vi "LJStreamM.vi"() -> ()   [LabVIEW 2026]
uses:
  Common Logger Controls/Currently Opened Device Params.ctl
  Common Logger Controls/Device Open Config Cluster.ctl
  Common Logger Controls/Channel Setup.ctl
  Common Logger Controls/Row Modification Options.ctl
  Common Logger Controls/Program Config Cluster.ctl
  sub/LJStreamM Front Panel References.ctl
  Common Logger VIs/LJM logger Globals.vi
panel:
  in  "Channel Setup":T1={"Name"=["AIN0", "AIN1", "AIN2", "AIN3", "AIN4", "AIN5", "AIN6", "AIN7", "AIN8", "AIN9", "AIN10", "AIN11", "AIN12", "AIN13", "AIN14", "AIN15", "AIN16", "AIN17", "AIN18", "AIN19", "AIN20", "AIN21", "AIN22", "AIN23", "AIN24", "AIN25", "AIN26", "AIN27", "AIN28", "AIN29", "AIN30", "AIN31", "AIN32", "AIN33", "AIN34", "AIN35", "AIN36", "AIN37", "AIN38", "AIN39", "AIN40", "AIN41", "AIN42", "AIN43", "AIN44", "AIN45", "AIN46", "AIN47", "AIN48", "AIN49", "AIN50", "AIN51", "AIN52", "AIN53", "AIN54", "AIN55", "AIN56", "AIN57", "AIN58", "AIN59", "AIN60", "AIN61", "AIN62", "AIN63", "AIN64", "AIN65", "AIN66", "AIN67", "AIN68", "AIN69", "AIN70", "AIN71", "AIN72", "AIN73", "AIN74", "AIN75", "AIN76", "AIN77", "AIN78", "AIN79", "AIN80", "AIN81", "AIN82", "AIN83", "AIN84", "AIN85", "AIN86", "AIN87", "AIN88", "AIN89", "AIN90", "AIN91", "AIN92", "AIN93", "AIN94", "AIN95", "AIN96", "AIN97", "AIN98", "AIN99"], "", "Scaling Equation"=["y=a", "y=b", "y=c", "y=d", "y=e", "y=f", "y=g", "y=h", "y=i", "y=j", "y=k", "y=l", "y=m", "y=n", "y=o", "y=p", "y=q", "y=r", "y=s", "y=t", "y=u", "y=v", "y=w", "y=x", "y=y", "y=z", "y=a2", "y=b2", "y=c2", "y=d2", "y=e2", "y=f2", "y=g2", "y=h2", "y=i2", "y=j2", "y=k2", "y=l2", "y=m2", "y=n2", "y=o2", "y=p2", "y=q2", "y=r2", "y=s2", "y=t2", "y=u2", "y=v2", "y=w2", "y=x2", "y=y2", "y=z2", "y=a3", "y=b3", "y=c3", "y=d3", "y=e3", "y=f3", "y=g3", "y=h3", "y=i3", "y=j3", "y=k3", "y=l3", "y=m3", "y=n3", "y=o3", "y=p3", "y=q3", "y=r3", "y=s3", "y=t3", "y=u3", "y=v3", "y=w3", "y=x3", "y=y3", "y=z3", "y=a4", "y=b4", "y=c4", "y=d4", "y=e4", "y=f4", "y=g4", "y=h4", "y=i4", "y=j4", "y=k4", "y=l4", "y=m4", "y=n4", "y=o4", "y=p4", "y=q4", "y=r4", "y=s4", "y=t4", "y=u4", "y=v4"], "", "Graph?"=[TRUE, TRUE, TRUE, TRUE, FALSE, FALSE, FALSE, FALSE, FALSE, FALSE, FALSE, FALSE, FALSE, FALSE, FALSE, FALSE]}
  in  "Stop Stream":bool
  out "Open Configs":T2
  out "Currently Opened Device Params":T3={"Device Type"="ANY", "Connection Type"="ANY", "Serial Number"=0}
  out "Program Config Name":string
  out "Open Config Name":string
  in  "Configuration":bool
  out "LJMScanBacklog":dbl format="%.2f"
  out "DeviceScanBacklog":dbl format="%.2f"
  in  "Disable Scaling*":bool=TRUE
  out "ms Per Loop":u32
  out "Scans Per Iteration":u32
  out "Iteration Number":i32
  out "Last Command-Response Error Message":string="No Error"
  in  "Max File Size (Bytes)":i32=1048576 min=1 max=2000000000
  out "Scaled Value":dbl[](array[numeric]) format="%.6f"
  out "Raw Value":dbl[](array[numeric]) format="%.6f"
  in  "Log To File":bool
  in  "exit":bool
  in  "# Scans On Graph":i32=1000 min=0
  in  "# Channels":i32=1 min=1 max=96
  out "Waveform Graph":cluster{dbl, dbl, dbl[][]}(graph)={0.0, 0.0025, []}
  in  "Scan Rate (Hz)":dbl=100.0 format="%.3f"
  out "Current Data File":path=path "Not Logging To File"
  in  "Data File Prefix":string="data"
  in  "start stream":bool caption="Start Stream"
  out "Last Stream Error Message":string="No Error"
  out "App Name":string
  in  "Row Modification Options":T4 {"Row #" min=0 max=95}
  # "Graph?"
  # "Name"
  # "Raw Value"
  # "Scaling Equation"
  # "Scaled Value"
  # "The raw value for each row corresponds to a scaling variable:"
  # "row 0-15   -->  \"a\"-\"p\""
  # "row 16-31 -->  \"a2\"-\"p2\""
  # "row 32-47 -->  \"a3\"-\"p3\""
  # "row 48-63 -->  \"a4\"-\"p4\""
  # "row 64-79 -->  \"a5\"-\"p5\""
  # "row 80-96 -->  \"a6\"-\"p6\""
  # "The scaled value for a row is represented by the variable  \"y\" in the row's scaling equation."
  # "If your scaling  equation has an error, the scaled value will be zero."
  # "*Scaling is computing intensive. If the LJM Backlog is growing, disable scaling."
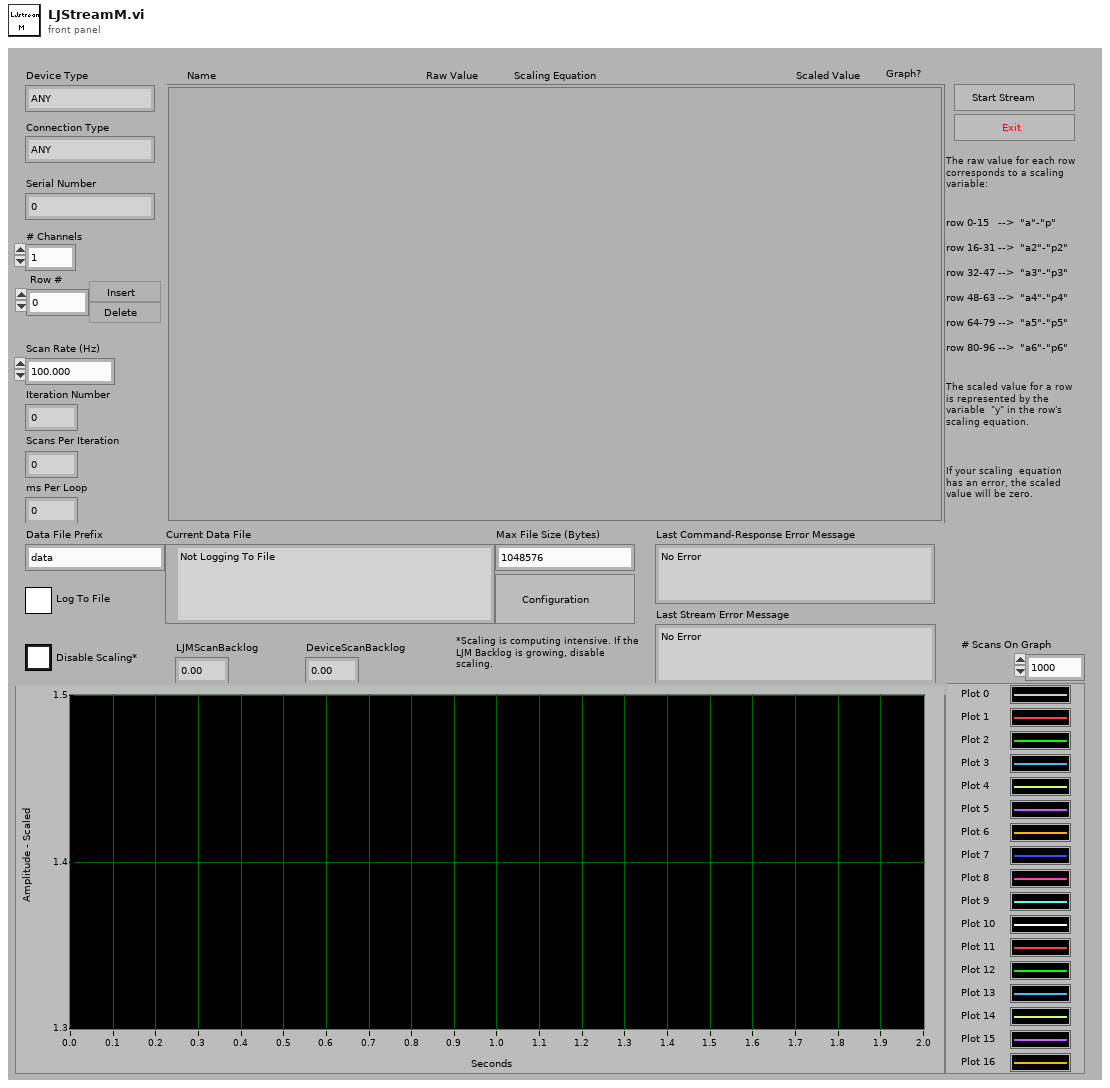
[diagram p1: front panel]
types:
  T1 = typedef "Channel Setup.ctl" = cluster{"Name":string[], string, "Scaling Equation":string[], string, "Graph?":bool[]}
  T2 = typedef "Device Open Config Cluster.ctl" = cluster{"Open Config Device Type":string, "Open Config Connection Type":string, "Open Config Identifier":string}
  T3 = typedef "Currently Opened Device Params.ctl" = cluster{"Device Type":string, "Connection Type":string, "Serial Number":i32}
  T4 = typedef "Row Modification Options.ctl" = cluster{" Row #":i32, "Delete Row":bool, "Insert Row":bool}
  T5 = typedef "LJStreamM Front Panel References.ctl" = cluster{"# Scans Read":refnum<vi>, "# of iterations Ref":refnum<vi>, "ms Per Loop Ref":refnum<vi>, "DeviceScanBacklog Ref":refnum<vi>, "LJMScanBacklog Ref":refnum<vi>, "Stop Stream Ref":refnum<vi>, "Disable Scaling* Ref":refnum<vi>, "Write To File Ref":refnum<vi>, "Current Data File Ref":refnum<vi>, "Waveform Graph Ref":refnum<vi>, "Data File Prefix Ref":refnum<vi>, "Max File Size (Bytes) Ref":refnum<vi>, "Channel Setup Reference In":refnum<vi>}
  T6 = typedef "Program Config Cluster.ctl" = cluster{"Data File Prefix":string, "Scan Rate (Hz)":dbl, "Graph History":i32, "# Channels":i32, "Disable Scaling":bool, "Max File Size (Bytes)":i32, "Channel Setup":T1, "Interval (ms)":u32, "Write To File":bool, "Log Every n Scans":i32}
  T7 = enum16{"Initialization", "Data Acquisition", "Shutdown", "Reconfiguration"}
  T8 = cluster{"Name":string[], string, "Scaling Equation":string[], string, "Graph?":bool[]}
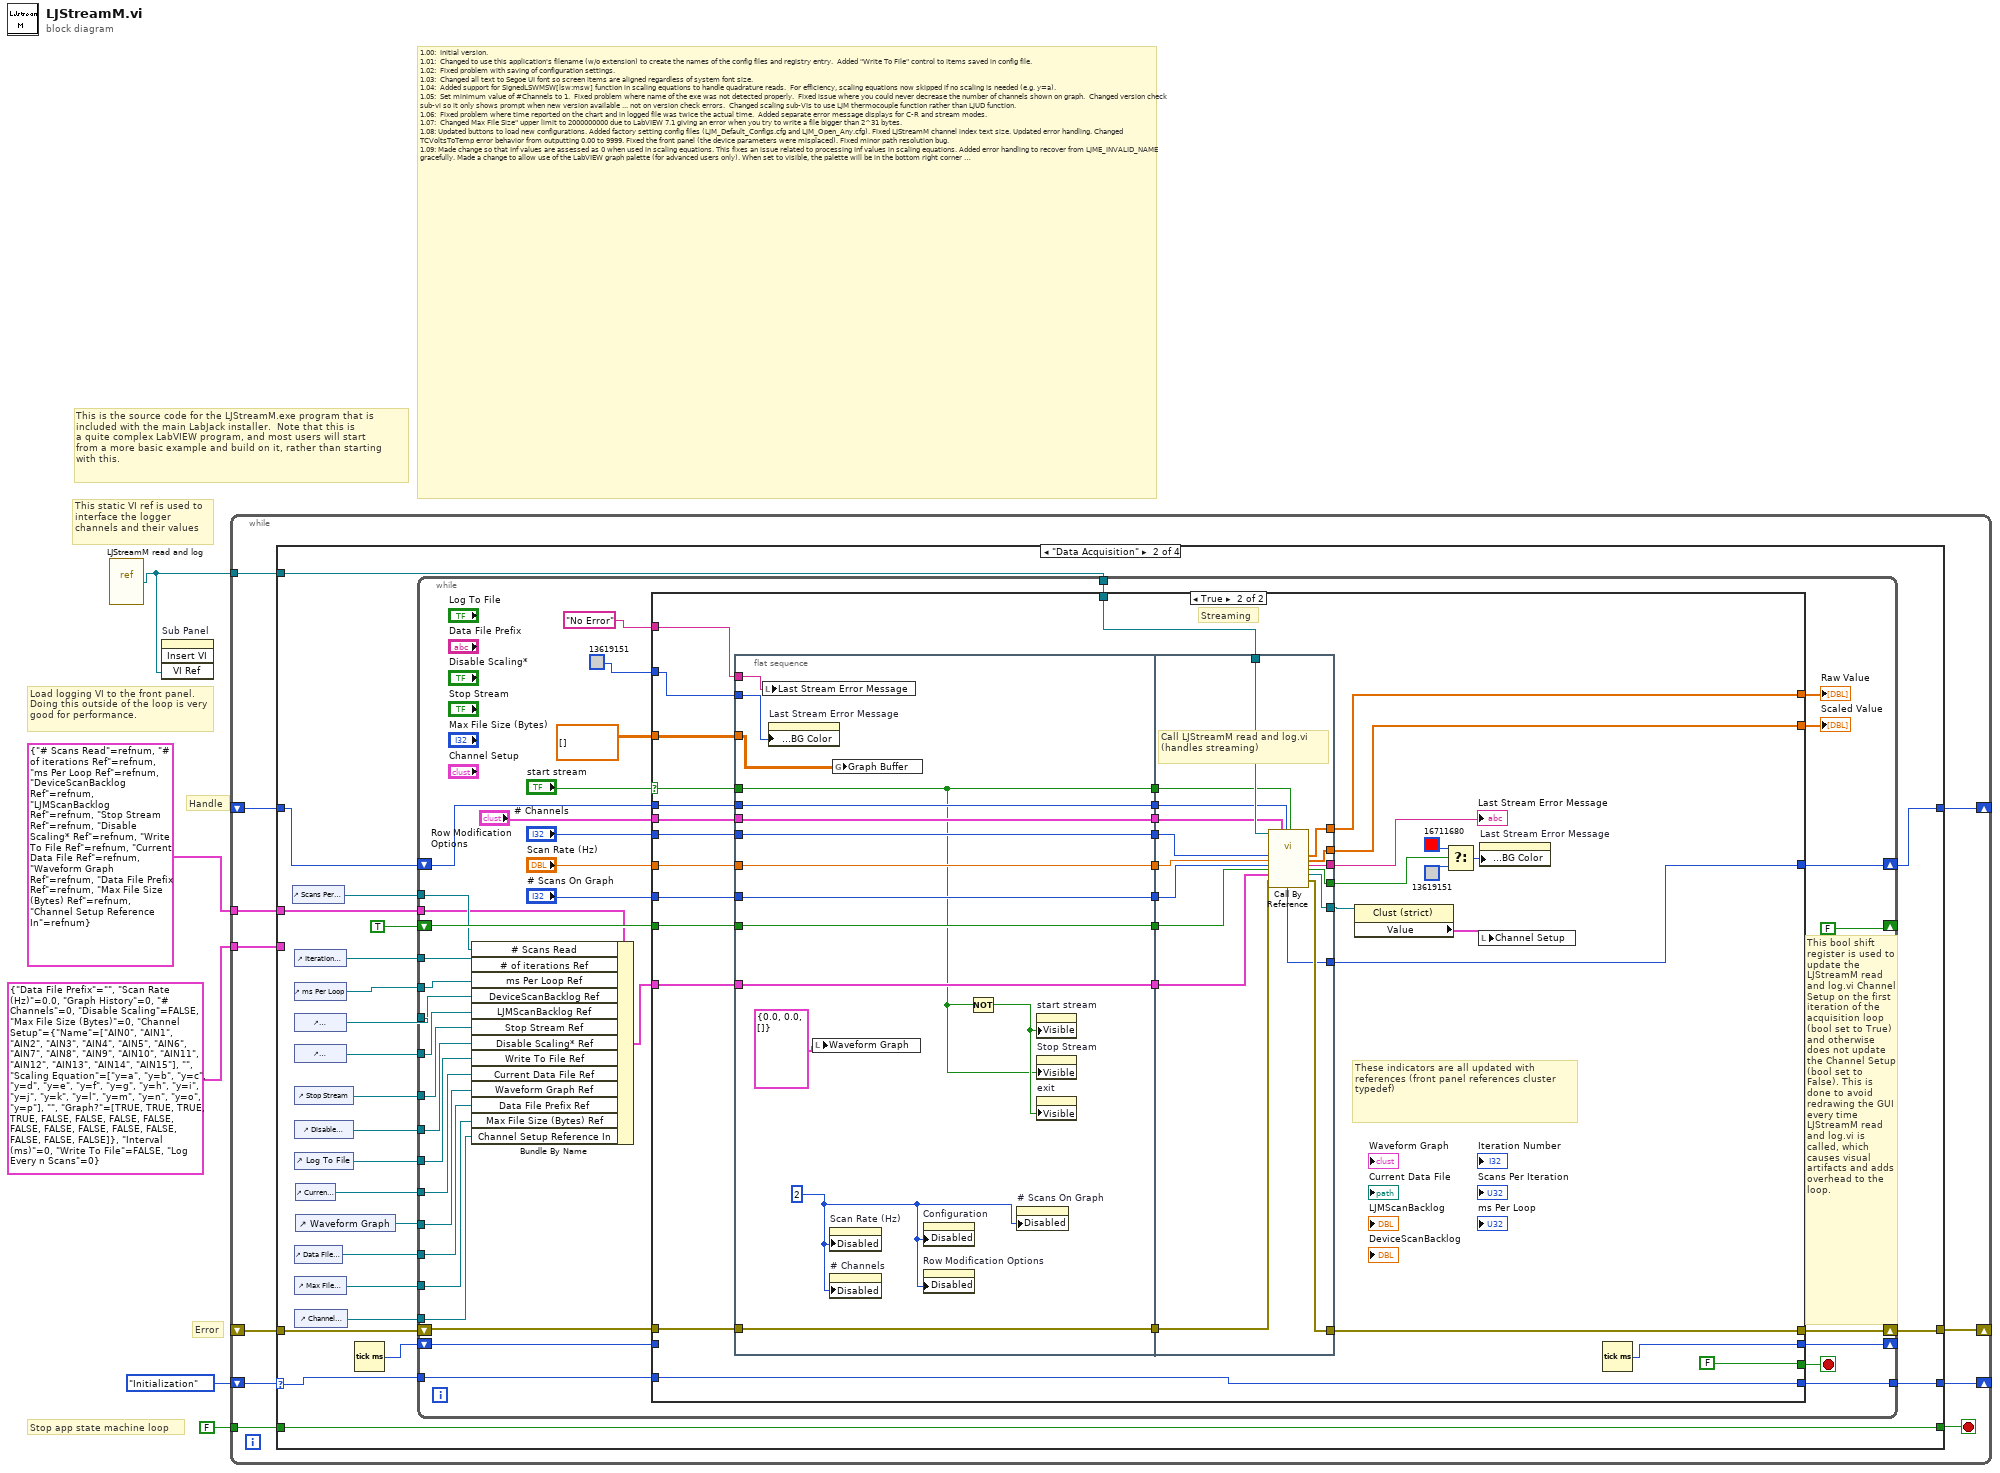
[diagram p0: block diagram]
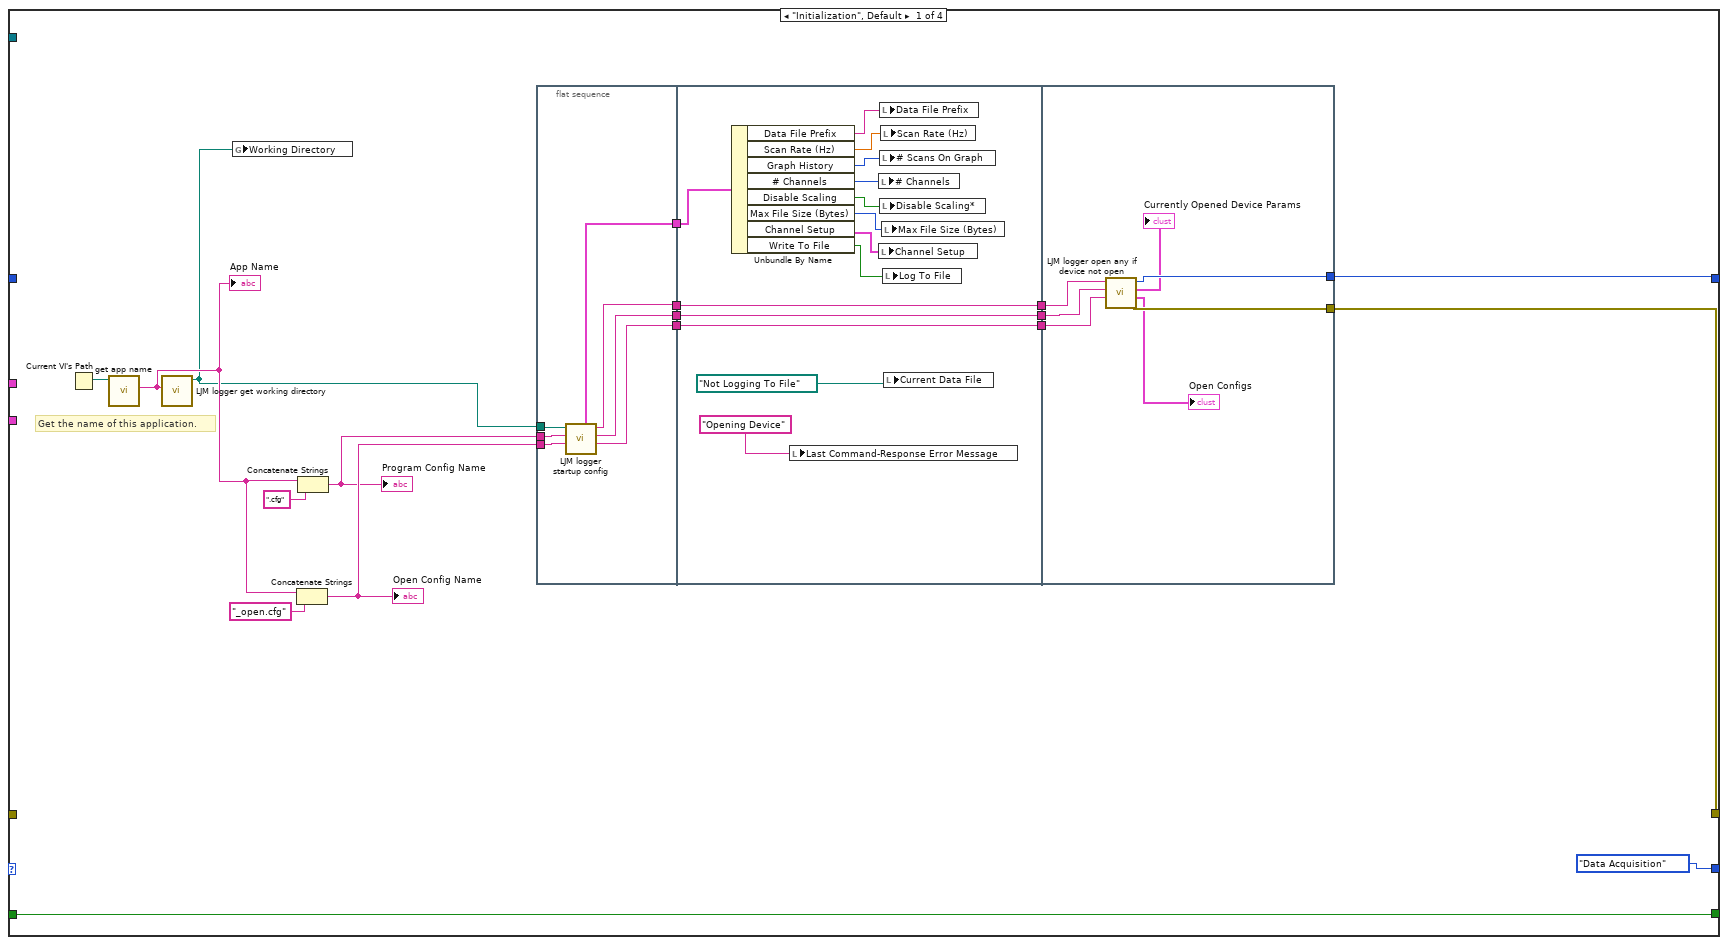
[diagram p2: hidden frame]
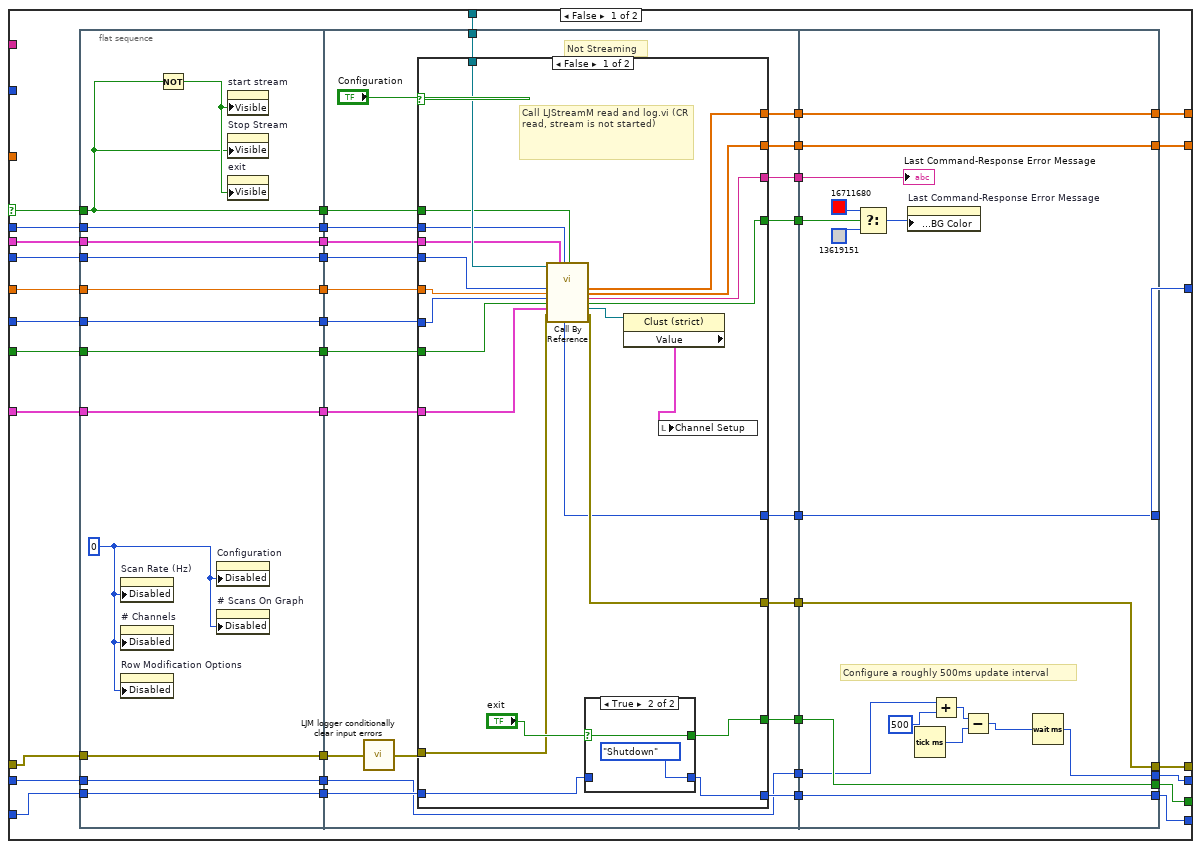
[diagram p3: hidden frame]
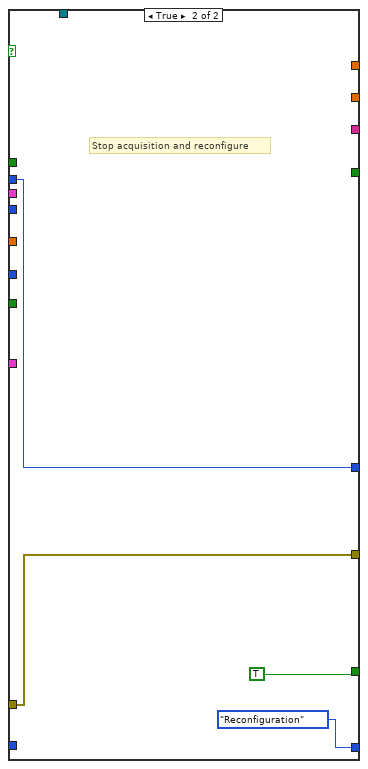
[diagram p5: hidden frame]
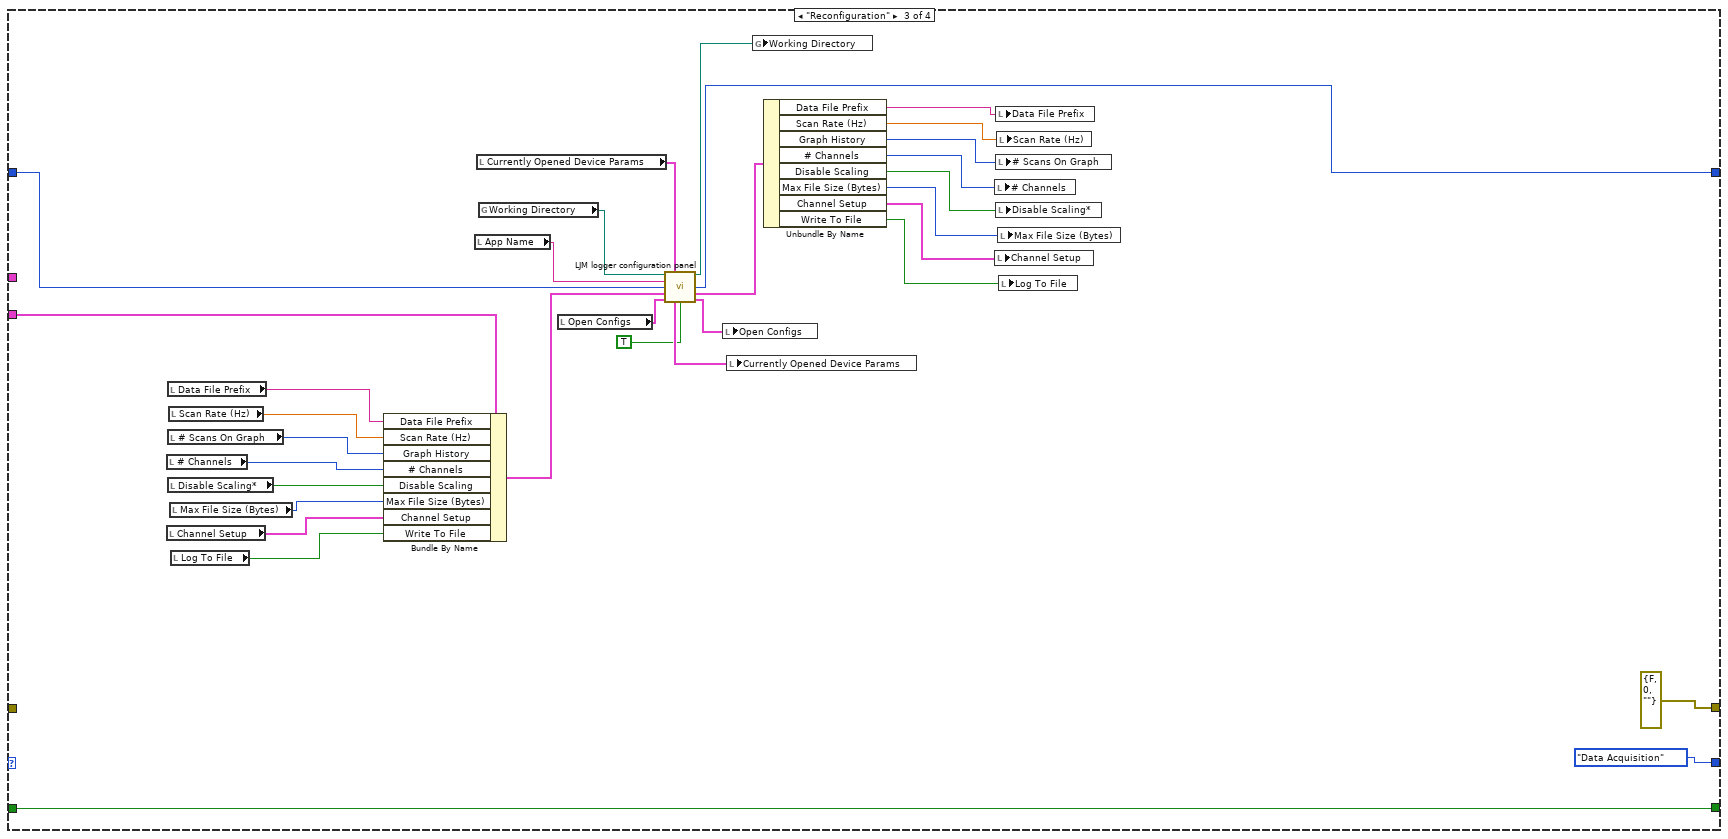
[diagram p6: hidden frame]
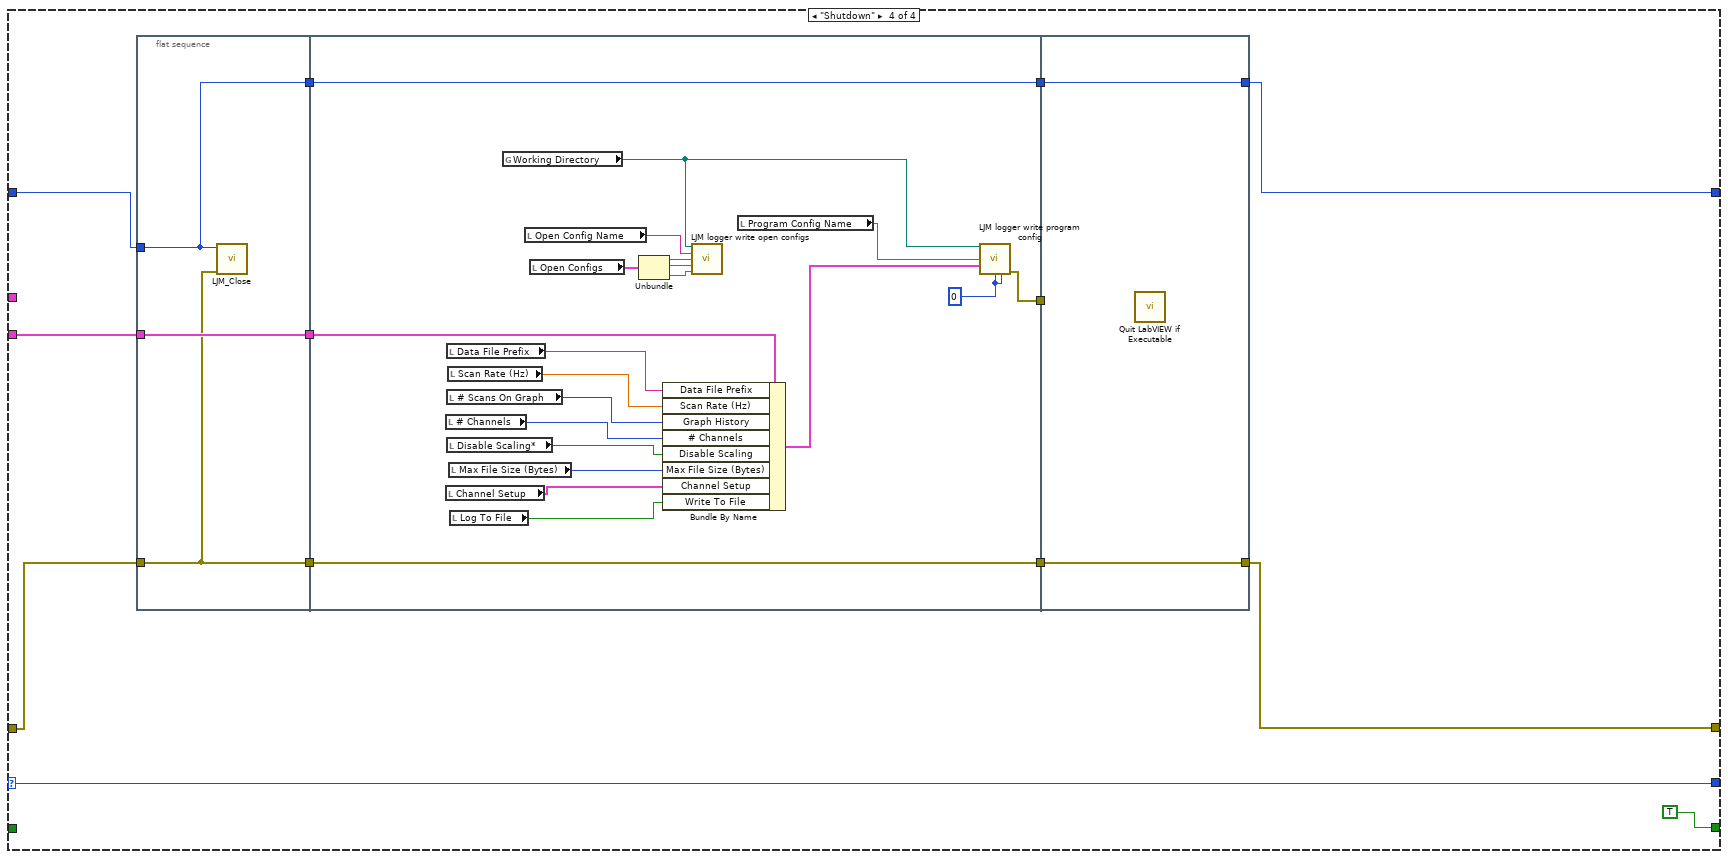
[diagram p7: hidden frame]
diagram:
  # "This static VI ref is used to interface the logger channels and their values"
  # "Load logging VI to the front panel. Doing this outside of the loop is very good for performance."
  # "Stop app state machine loop"
  # "Error"
  # "Handle"
  # "This is the source code for the LJStreamM.exe program that is\nincluded with the main LabJack installer.  Note that this is \na quite complex LabVIEW program, and most users will start\nfrom a more basic example and build on it, rather than starting\nwith this."
  # "1.00:  Initial version.\n1.01:  Changed to use this application's filename (w/o extension) to create the names of the config files and registry entry.  Added \"Write To File\" control to items saved in config file.\n1.02:  Fixed problem with saving of configuration settings.\n1.03:  Changed all text to Segoe UI font so screen items are aligned regardless of system font size.\n1.04:  Added support for SignedLSWMSW[lsw:msw] function in scaling equations to handle quadrature reads.  For efficiency, scaling equations now skipped if no scaling is needed (e.g. y=a).\n1.05:  Set minimum value of #Channels to 1.  Fixed problem where name of the exe was not detected properly.  Fixed issue where you could never decrease the number of channels shown on graph.  Changed version check sub-vi so it only shows prompt when new version available ... not on version check errors.  Changed scaling sub-VIs to use LJM thermocouple function rather than LJUD function.\n1.06:  Fixed problem where time reported on the chart and in logged file was twice the actual time.  Added separate error message displays for C-R and stream modes.\n1.07:  Changed Max File Size\" upper limit to 2000000000 due to LabVIEW 7.1 giving an error when you try to write a file bigger than 2^31 bytes.\n1.08: Updated buttons to load new configurations. Added factory setting config files (LJM_Default_Configs.cfg and LJM_Open_Any.cfg). Fixed LJStreamM channel index text size. Updated error handling. Changed TCVoltsToTemp error behavior from outputting 0.00 to 9999. Fixed the front panel (the device parameters were misplaced). Fixed minor path resolution bug.\n1.09: Made change so that Inf values are assessed as 0 when used in scaling equations. This fixes an issue related to processing Inf values in scaling equations. Added error handling to recover from LJME_INVALID_NAME gracefully. Made a change to allow use of the LabVIEW graph palette (for advanced users only). When set to visible, the palette will be in the bottom right corner of the LJStreamM graph. \n1.10: Fixed SignedMSWLSW scaling equation functionality. This was previously returning an unsigned 32-bit integer representation. It now returns a signed 32-bit integer representation.\n1.11: Reworked configs including adding a config panel. Moved 'Change Working Directory'. Refactored write to file functionality. Refactored diagram. Added scaling equation error messaging. Renamed 'experiment' config 'program' config. Added register write functionality to configuration panel. Increased front panel text size, changed font to Arial (monospace), and set the minimum panel size. Added support for 96 channels.  Added logger row modification controls. Note: program configs with 96 channels in v1.11 would not be recognized as valid in v1.10.\n1.12: Made minor Visual tweaks to the front panel. Made optimizations to scaling equation processing and front panel responsiveness. Disabled the scaling equation control while stream is active.\n1.13: If a config file does not exist, load defaults without warning the user. Usually if the config file does not exist it means this is the first time running the program, and we do not want new users to see a warning about the config not existing. Rearranged logger graph palettes on the front panel"
  n1 = vi-ref "LJStreamM read and log.vi"() -> ("vi reference"=w2:refnum<vi>)
  n2 = invoke on="Sub Panel" class="SubPanel" method="Insert VI"("VI Ref"=w2) -> ()  [unwired: 3 in, 4 out]
  n3 = while {
    shift-right: [w14] -> _
    shift-left: _ -> [w11]
    shift-right: [w15] -> _
    shift-left: _ -> [w12]
    shift-right: [w13] -> _
    shift-left: T7."Initialization" -> [w16]
    tunnel: T6 {"Data File Prefix"="", "Scan Rate (Hz)"=0.0, "Graph History"=0, "# Channels"=0, "Disable Scaling"=FALSE, "Max File Size (Bytes)"=0, "Channel Setup"={"Name"=["AIN0", "AIN1", "AIN2", "AIN3", "AIN4", "AIN5", "AIN6", "AIN7", "AIN8", "AIN9", "AIN10", "AIN11", "AIN12", "AIN13", "AIN14", "AIN15"], "", "Scaling Equation"=["y=a", "y=b", "y=c", "y=d", "y=e", "y=f", "y=g", "y=h", "y=i", "y=j", "y=k", "y=l", "y=m", "y=n", "y=o", "y=p"], "", "Graph?"=[TRUE, TRUE, TRUE, TRUE, FALSE, FALSE, FALSE, FALSE, FALSE, FALSE, FALSE, FALSE, FALSE, FALSE, FALSE, FALSE]}, "Interval (ms)"=0, "Write To File"=FALSE, "Log Every n Scans"=0} ("Program Configs") -> [w10]
    tunnel: FALSE -> [w8]
    tunnel: w2 -> [w7]
    tunnel: T5 {"# Scans Read"=refnum, "# of iterations Ref"=refnum, "ms Per Loop Ref"=refnum, "DeviceScanBacklog Ref"=refnum, "LJMScanBacklog Ref"=refnum, "Stop Stream Ref"=refnum, "Disable Scaling* Ref"=refnum, "Write To File Ref"=refnum, "Current Data File Ref"=refnum, "Waveform Graph Ref"=refnum, "Data File Prefix Ref"=refnum, "Max File Size (Bytes) Ref"=refnum, "Channel Setup Reference In"=refnum} ("LJStreamM Front Panel References") -> [w6]
    stop <- w9 stop-if-true
    n4 = case shown="\"Data Acquisition\"" w16 {
      selector: w16 -> [_ w69 _ w357]
      tunnel: [w20 w84 w343 w347] -> w15
      tunnel: [w19 w83 errorcluster {"status"=FALSE, "code"=0, "source"=""} ("error out") w346] -> w14
      tunnel: [T7."Data Acquisition" w85 T7."Data Acquisition" w357] -> w13
      tunnel: w12 -> [_ w81 w342 w353]
      tunnel: w11 -> [_ w82 _ w352]
      tunnel: w10 -> [_ _ w340 w356]
      tunnel: [w17 w86 w339 TRUE] -> w9
      tunnel: w8 -> [w17 w86 w339 _]
      tunnel: w7 -> [_ w80 _ _]
      tunnel: w6 -> [_ w68 _ _]
      frame "Initialization", Default {
        # "Get the name of this application."
        n5 = Current VI's Path() -> (path=w21:path)
        n6 = call "get app name.vi"("Current VI's Path"=w21) -> ("App Name Without Extension"=w25:string)  [unwired: 4 in, 2 out]
        "App Name" <- w25
        n7 = call "LJM logger get working directory.vi"("Application Name"=w25) -> ("Working Directory"=w22:path)  [unwired: 9 in, 1 out]
        n8 = global write "LJM logger Globals.vi" "Working Directory"(w22) -> ()
        n9 = Concatenate Strings(w25, "_open.cfg" ("string")) -> (w27:string)
        "Open Config Name" <- w27
        n10 = Concatenate Strings(w25, ".cfg" ("string")) -> (w26:string)
        "Program Config Name" <- w26
        n11 = flat-sequence {
          tunnel: [w40] -> w34
          tunnel: [w39] -> w33
          tunnel: [w38] -> w32
          tunnel: w22 -> [w41]
          tunnel: w26 -> [w37]
          tunnel: w27 -> [w36]
          tunnel: [w35] -> w31
          tunnel: w34 -> [w55]
          tunnel: w33 -> [w54]
          tunnel: w32 -> [w53]
          tunnel: [w55] -> w30
          tunnel: [w54] -> w29
          tunnel: [w53] -> w28
          tunnel: w31 -> [w52]
          tunnel: w30 -> [w62]
          tunnel: w29 -> [w61]
          tunnel: w28 -> [w60]
          tunnel: [w58] -> w19
          tunnel: [w59] -> w20
          frame #0 {
            n12 = call "LJM logger startup config.vi"("Device Open Config Name"=w36, "Program Config Name"=w37, "Working Directory"=w41) -> ("Open Config Identifier"=w38:string, "Open Config ConnectionType"=w39:string, "Open Config Device Type"=w40:string, "Program Configs"=w35:T6)  [unwired: 3 in]
          }
          frame #1 {
            n13 = Unbundle By Name(w52) -> ("Data File Prefix"=w51:string, "Scan Rate (Hz)"=w50:dbl, "Graph History"=w49:i32, "# Channels"=w48:i32, "Disable Scaling"=w47:bool, "Max File Size (Bytes)"=w46:i32, "Channel Setup"=w44:T1, "Write To File"=w45:bool)
            n14 = local write "Last Command-Response Error Message"("Opening Device" ("source")) -> ()
            n15 = local write "# Channels"(w48) -> ()
            n16 = local write "Channel Setup"(w44) -> ()
            n17 = local write "Data File Prefix"(w51) -> ()
            n18 = local write "# Scans On Graph"(w49) -> ()
            n19 = local write "Disable Scaling*"(w47) -> ()
            n20 = local write "Scan Rate (Hz)"(w50) -> ()
            n21 = local write "Max File Size (Bytes)"(w46) -> ()
            n22 = local write "Log To File"(w45) -> ()
            n23 = local write "Current Data File"(path "Not Logging To File" ("Current Data File")) -> ()
          }
          frame #2 {
            n24 = call "LJM logger open any if device not open.vi"("Open Config Identifier"=w60, "Open Config Connection Type"=w61, "Open Config DeviceType"=w62) -> ("error out"=w58:errorcluster, "Open Configs"=→"Open Configs":T2, "Currently Opened Device Params"=→"Currently Opened Device Params":T3, "Handle Out"=w59:i32)  [unwired: 5 in]
          }
        }
      }
      frame "Data Acquisition" {
        n25 = control-ref of="Scans Per Iteration"() -> (w79:refnum<vi>)
        n26 = control-ref of="Iteration Number"() -> (w78:refnum<vi>)
        n27 = control-ref of="ms Per Loop"() -> (w77:refnum<vi>)
        n28 = control-ref of="DeviceScanBacklog"() -> (w76:refnum<vi>)
        n29 = control-ref of="LJMScanBacklog"() -> (w75:refnum<vi>)
        n30 = control-ref of="Stop Stream"() -> (w74:refnum<vi>)
        n31 = control-ref of="Disable Scaling*"() -> (w73:refnum<vi>)
        n32 = control-ref of="Log To File"() -> (w72:refnum<vi>)
        n33 = control-ref of="Data File Prefix"() -> (w67:refnum<vi>)
        n34 = control-ref of="Max File Size (Bytes)"() -> (w66:refnum<vi>)
        n35 = control-ref of="Channel Setup"() -> (w65:refnum<vi>)
        n36 = control-ref of="Current Data File"() -> (w71:refnum<vi>)
        n37 = control-ref of="Waveform Graph"() -> (w70:refnum<vi>)
        n38 = Tick Count (ms)() -> (millisecond timer value=w63:u32)
        n39 = while {
          shift-right: [w93] -> w84
          shift-left: w81 -> [w110]
          shift-right: [w114] -> w83
          shift-left: w82 -> [w111]
          tunnel: w80 -> [w116]
          shift-right: [FALSE] -> _
          shift-left: TRUE -> [w115]
          tunnel: [w108] -> w85
          tunnel: w79 -> [w106]
          tunnel: w78 -> [w105]
          tunnel: w77 -> [w104]
          tunnel: w76 -> [w103]
          tunnel: w75 -> [w102]
          tunnel: w74 -> [w101]
          tunnel: w73 -> [w100]
          tunnel: w72 -> [w99]
          tunnel: w71 -> [w98]
          tunnel: w70 -> [w97]
          tunnel: w69 -> [w109]
          tunnel: w68 -> [w96]
          tunnel: w67 -> [w95]
          tunnel: w66 -> [w94]
          tunnel: w65 -> [w91]
          shift-right: [w88] -> _
          shift-left: w63 -> [w87]
          stop <- w107 stop-if-true
          # "This bool shift register is used to update the LJStreamM read and log.vi Channel Setup on the first iteration of the acquisition loop (bool set to True) and otherwise does not update the Channel Setup (bool set to False). This is done to avoid redrawing the GUI every time LJStreamM read and log.vi is called, which causes visual artifacts and adds overhead to the loop."
          n40 = Bundle By Name(cluster=w96, "# Scans Read"=w106, "# of iterations Ref"=w105, "ms Per Loop Ref"=w104, "DeviceScanBacklog Ref"=w103, "LJMScanBacklog Ref"=w102, "Stop Stream Ref"=w101, "Disable Scaling* Ref"=w100, "Write To File Ref"=w99, "Current Data File Ref"=w98, "Waveform Graph Ref"=w97, "Data File Prefix Ref"=w95, "Max File Size (Bytes) Ref"=w94, "Channel Setup Reference In"=w91) -> (w92:T5)
          n41 = case shown="True" "start stream" {
            selector: "start stream" -> [w157 w272]
            tunnel: dbl[][] [] ("Graph Buffer") -> [_ w253]
            tunnel: u32 13619151 -> [_ w254]
            tunnel: "No Error" ("Last Stream Error Message") -> [_ w255]
            tunnel: "# Scans On Graph" -> [w161 w276]
            tunnel: "# Channels" -> [w159 w274]
            tunnel: "Scan Rate (Hz)" -> [w160 w275]
            tunnel: w116 -> [w162 w256]
            tunnel: w115 -> [w153 w268]
            tunnel: w110 -> [w158 w273]
            tunnel: w111 -> [w155 w277]
            tunnel: [w156 w271] -> w114
            tunnel: [w135 w267] -> w113
            tunnel: [w137 w266] -> w112
            tunnel: [w154 w264] -> w108
            tunnel: w109 -> [w152 w264]
            tunnel: [w151 FALSE] -> w107
            tunnel: [w130 w250] -> w93
            tunnel: w92 -> [w139 w248]
            tunnel: "Row Modification Options" -> [w129 w247]
            tunnel: [w127 w245] -> w88
            tunnel: w87 -> [w124 _]
            frame False {
              n42 = flat-sequence {
                tunnel: w152 -> [w169]
                tunnel: w153 -> [w170]
                tunnel: w155 -> [w171]
                tunnel: w157 -> [w165]
                tunnel: w158 -> [w172]
                tunnel: w159 -> [w173]
                tunnel: w160 -> [w174]
                tunnel: w161 -> [w175]
                tunnel: [w175] -> w147
                tunnel: [w174] -> w146
                tunnel: [w173] -> w145
                tunnel: [w172] -> w144
                tunnel: [w165] -> w143
                tunnel: [w171] -> w142
                tunnel: [w170] -> w141
                tunnel: [w169] -> w140
                tunnel: w139 -> [w168]
                tunnel: [w168] -> w138
                tunnel: w129 -> [w167]
                tunnel: [w167] -> w128
                tunnel: w124 -> [w163]
                tunnel: [w163] -> w125
                tunnel: w162 -> [w197]
                tunnel: [w190] -> w150
                tunnel: [w187] -> w149
                tunnel: [w184] -> w148
                tunnel: w147 -> [w195]
                tunnel: w146 -> [w194]
                tunnel: w145 -> [w193]
                tunnel: w144 -> [w192]
                tunnel: w143 -> [w191]
                tunnel: w142 -> [w189]
                tunnel: w141 -> [w186]
                tunnel: w140 -> [w185]
                tunnel: w138 -> [w183]
                tunnel: [w182] -> w136
                tunnel: [w181] -> w134
                tunnel: [w180] -> w133
                tunnel: [w179] -> w132
                tunnel: [w178] -> w131
                tunnel: w128 -> [w177]
                tunnel: w125 -> [w176]
                tunnel: [w176] -> w126
                tunnel: [w242] -> w151
                tunnel: [w243] -> w154
                tunnel: [w244] -> w156
                tunnel: w150 -> [w244]
                tunnel: w149 -> [w243]
                tunnel: w148 -> [w242]
                tunnel: [w238] -> w137
                tunnel: w136 -> [w238]
                tunnel: [w237] -> w135
                tunnel: w134 -> [w237]
                tunnel: w133 -> [w236]
                tunnel: w132 -> [w235]
                tunnel: w131 -> [w234]
                tunnel: [w234] -> w130
                tunnel: [w233] -> w127
                tunnel: w126 -> [w228]
                frame #0 {
                  w164 = u8 0 ("Disabled")
                  n43 = property on="Scan Rate (Hz)" class="DigNum (strict)"("Disabled"=w164) -> ()  [unwired: 2 in, 2 out]
                  n44 = property on="# Channels" class="DigNum (strict)"("Disabled"=w164) -> ()  [unwired: 2 in, 2 out]
                  n45 = property on="Row Modification Options" class="Clust"("Disabled"=w164) -> ()  [unwired: 2 in, 2 out]
                  n46 = Not(x=w165) -> (.not. x?=w166:bool)
                  n47 = property on="Configuration" class="Bool"("Disabled"=w164) -> ()  [unwired: 2 in, 2 out]
                  n48 = property on="# Scans On Graph" class="DigNum (strict)"("Disabled"=w164) -> ()  [unwired: 2 in, 2 out]
                  n49 = property on="start stream" class="Bool"("Visible"=w166) -> ()  [unwired: 2 in, 2 out]
                  n50 = property on="Stop Stream" class="Bool (strict)"("Visible"=w165) -> ()  [unwired: 2 in, 2 out]
                  n51 = property on="exit" class="Bool"("Visible"=w166) -> ()  [unwired: 2 in, 2 out]
                }
                frame #1 {
                  # "Not Streaming"
                  n52 = call "LJM logger conditionally clear input errors.vi"("error in"=w189) -> ("error out"=w188:errorcluster)
                  n53 = case shown="False" "Configuration" {
                    tunnel: [w217 T7."Reconfiguration"] -> w187
                    tunnel: w197 -> [w214 _]
                    tunnel: w188 -> [w207 w226]
                    tunnel: [w201 w226] -> w190
                    tunnel: w186 -> [w199 _]
                    tunnel: w195 -> [w209 _]
                    tunnel: w194 -> [w210 _]
                    tunnel: w193 -> [w211 _]
                    tunnel: w192 -> [w212 w224]
                    tunnel: w191 -> [w213 _]
                    tunnel: w185 -> [w218 _]
                    tunnel: [w216 TRUE] -> w184
                    tunnel: w183 -> [w208 _]
                    tunnel: [w206 _] -> w182
                    tunnel: [w205 _] -> w181
                    tunnel: [w204 _] -> w180
                    tunnel: [w203 _] -> w179
                    tunnel: [w200 w224] -> w178
                    tunnel: w177 -> [w198 _]
                    frame False {
                      # "Call LJStreamM read and log.vi (CR read, stream is not started)"
                      n54 = call-by-ref "?"(reference=w214, "# Channels"=w211, "Scan Rate (Hz)"=w210, "# Scans On Graph"=w209, "Update Channel Ref"=w199, "LJStreamM Front Panel References"=w208, "(LJM) Error In"=w207, "Row Modification Options"=w198, "Handle In"=w212, "start stream"=w213) -> ("Handle Out"=w200:i32, "Raw Value"=w206:dbl[], "Scaled Value"=w205:dbl[], "Last Error Message"=w204:string, "Last Error Message Status"=w203:bool, "Channel Setup Reference Out"=w202:refnum<vi>, "(LJM) Error Out"=w201:errorcluster)  [unwired: 5 in, 2 out]
                      n55 = case shown="True" "exit" {
                        selector: "exit" -> [w221 w222]
                        tunnel: [w220 T7."Shutdown"] -> w217
                        tunnel: [w221 w222] -> w216
                        tunnel: w218 -> [w220 _]
                        frame False {
                        }
                        frame True {
                        }
                      }
                      n56 = property on="Property Node" class="Clust (strict)"(reference=w202) -> ("Value"=w215:T8)  [unwired: 1 in, 2 out]
                      n57 = local write "Channel Setup"(w215) -> ()
                    }
                    frame True {
                      # "Stop acquisition and reconfigure"
                    }
                  }
                }
                frame #2 {
                  # "Configure a roughly 500ms update interval"
                  n58 = Select(t=u32 16711680, s=w235, f=u32 13619151) -> (s? t:f=w241:u32)
                  n59 = property on="Last Command-Response Error Message" class="Str"("Text.Text Colors:BG Color"=w241) -> ()  [unwired: 2 in, 2 out]
                  n60 = Tick Count (ms)() -> (millisecond timer value=w232:u32)
                  n61 = Add(x=w228, y=u16 500) -> (x+y=w230:u32)
                  n62 = Subtract(x=w230, y=w232) -> (x-y=w229:u32)
                  n63 = Wait (ms)(milliseconds to wait=w229) -> (millisecond timer value=w233:u32)
                  "Last Command-Response Error Message" <- w236
                }
              }
            }
            frame True {
              # "Streaming"
              # "These indicators are all updated with references (front panel references cluster typedef)"
              n64 = flat-sequence {
                tunnel: w268 -> [w290]
                tunnel: w272 -> [w282]
                tunnel: w273 -> [w291]
                tunnel: w274 -> [w292]
                tunnel: w275 -> [w293]
                tunnel: w276 -> [w294]
                tunnel: w277 -> [w295]
                tunnel: [w295] -> w263
                tunnel: [w294] -> w262
                tunnel: [w293] -> w261
                tunnel: [w292] -> w260
                tunnel: [w291] -> w259
                tunnel: [w282] -> w258
                tunnel: [w290] -> w257
                tunnel: w255 -> [w288]
                tunnel: w254 -> [w287]
                tunnel: w253 -> [w286]
                tunnel: w248 -> [w285]
                tunnel: [w285] -> w249
                tunnel: w247 -> [w284]
                tunnel: [w284] -> w246
                tunnel: [w310] -> w271
                tunnel: [w309] -> w270
                tunnel: [w305] -> w267
                tunnel: [w306] -> w266
                tunnel: w263 -> [w312]
                tunnel: w262 -> [w299]
                tunnel: w261 -> [w311]
                tunnel: w260 -> [w300]
                tunnel: w259 -> [w301]
                tunnel: w258 -> [w307]
                tunnel: w257 -> [w298]
                tunnel: w256 -> [w308]
                tunnel: [w304] -> w252
                tunnel: [w303] -> w251
                tunnel: [w302] -> w250
                tunnel: w249 -> [w297]
                tunnel: w246 -> [w296]
                frame #0 {
                  w281 = u8 2 ("Disabled")
                  n65 = local write "Last Stream Error Message"(w288) -> ()
                  n66 = property on="Last Stream Error Message" class="Str"("Text.Text Colors:BG Color"=w287) -> ()  [unwired: 2 in, 2 out]
                  n67 = local write "Waveform Graph"(cluster{dbl, dbl, dbl[][]} {0.0, 0.0, []} ("Waveform Graph")) -> ()
                  n68 = property on="Scan Rate (Hz)" class="DigNum (strict)"("Disabled"=w281) -> ()  [unwired: 2 in, 2 out]
                  n69 = property on="# Channels" class="DigNum (strict)"("Disabled"=w281) -> ()  [unwired: 2 in, 2 out]
                  n70 = global write "LJM logger Globals.vi" "Graph Buffer"(w286) -> ()
                  n71 = property on="Configuration" class="Bool"("Disabled"=w281) -> ()  [unwired: 2 in, 2 out]
                  n72 = property on="Row Modification Options" class="Clust"("Disabled"=w281) -> ()  [unwired: 2 in, 2 out]
                  n73 = Not(x=w282) -> (.not. x?=w283:bool)
                  n74 = property on="# Scans On Graph" class="DigNum (strict)"("Disabled"=w281) -> ()  [unwired: 2 in, 2 out]
                  n75 = property on="start stream" class="Bool"("Visible"=w283) -> ()  [unwired: 2 in, 2 out]
                  n76 = property on="Stop Stream" class="Bool (strict)"("Visible"=w282) -> ()  [unwired: 2 in, 2 out]
                  n77 = property on="exit" class="Bool"("Visible"=w283) -> ()  [unwired: 2 in, 2 out]
                }
                frame #1 {
                  # "Call LJStreamM read and log.vi (handles streaming)"
                  n78 = call-by-ref "?"(reference=w308, "# Channels"=w300, "Scan Rate (Hz)"=w311, "# Scans On Graph"=w299, "Update Channel Ref"=w298, "LJStreamM Front Panel References"=w297, "(LJM) Error In"=w312, "Row Modification Options"=w296, "Handle In"=w301, "start stream"=w307) -> ("Handle Out"=w302:i32, "Raw Value"=w306:dbl[], "Scaled Value"=w305:dbl[], "Last Error Message"=w303:string, "Last Error Message Status"=w304:bool, "Channel Setup Reference Out"=w309:refnum<vi>, "(LJM) Error Out"=w310:errorcluster)  [unwired: 5 in, 2 out]
                }
              }
              n79 = property on="Property Node" class="Clust (strict)"(reference=w270) -> ("Value"=w269:T8)  [unwired: 1 in, 2 out]
              n80 = Select(t=u32 16711680, s=w252, f=u32 13619151) -> (s? t:f=w278:u32)
              n81 = local write "Channel Setup"(w269) -> ()
              n82 = property on="Last Stream Error Message" class="Str"("Text.Text Colors:BG Color"=w278) -> ()  [unwired: 2 in, 2 out]
              n83 = Tick Count (ms)() -> (millisecond timer value=w245:u32)
              "Last Stream Error Message" <- w251
            }
          }
          "Raw Value" <- w112
          "Scaled Value" <- w113
        }
      }
      frame "Reconfiguration" {
        n84 = local read "# Channels"() -> (w319:i32)
        n85 = local read "Channel Setup"() -> (w316:T1)
        n86 = local read "Data File Prefix"() -> (w322:string)
        n87 = local read "# Scans On Graph"() -> (w320:i32)
        n88 = local read "Disable Scaling*"() -> (w318:bool)
        n89 = local read "Scan Rate (Hz)"() -> (w321:dbl)
        n90 = local read "Max File Size (Bytes)"() -> (w317:i32)
        n91 = local read "Log To File"() -> (w315:bool)
        n92 = Bundle By Name(cluster=w340, "Data File Prefix"=w322, "Scan Rate (Hz)"=w321, "Graph History"=w320, "# Channels"=w319, "Disable Scaling"=w318, "Max File Size (Bytes)"=w317, "Channel Setup"=w316, "Write To File"=w315) -> (w323:T6)
        n93 = local read "App Name"() -> (w338:string)
        n94 = local read "Currently Opened Device Params"() -> (w336:T3)
        n95 = global read "LJM logger Globals.vi" "Working Directory"() -> (w325:path)
        n96 = local read "Open Configs"() -> (w337:T2)
        n97 = call "LJM logger configuration panel.vi"("Working Directory"=w325, "Current Device Connection In"=w336, "App name"=w338, "Handle In"=w342, "Program Configs"=w323, "Device Open Params In"=w337, "Streaming App?"=TRUE) -> ("Working Directory Out"=w313:path, "Handle Out"=w343:i32, "Program Configs Out"=w324:T6, "Current Device Connection Out"=w335:T3, "Device Open Params Out"=w334:T2)  [unwired: 4 in]
        n98 = local write "Open Configs"(w334) -> ()
        n99 = local write "Currently Opened Device Params"(w335) -> ()
        n100 = global write "LJM logger Globals.vi" "Working Directory"(w313) -> ()
        n101 = Unbundle By Name(w324) -> ("Data File Prefix"=w333:string, "Scan Rate (Hz)"=w332:dbl, "Graph History"=w331:i32, "# Channels"=w330:i32, "Disable Scaling"=w329:bool, "Max File Size (Bytes)"=w328:i32, "Channel Setup"=w326:T1, "Write To File"=w327:bool)
        n102 = local write "# Channels"(w330) -> ()
        n103 = local write "Channel Setup"(w326) -> ()
        n104 = local write "Data File Prefix"(w333) -> ()
        n105 = local write "# Scans On Graph"(w331) -> ()
        n106 = local write "Disable Scaling*"(w329) -> ()
        n107 = local write "Scan Rate (Hz)"(w332) -> ()
        n108 = local write "Max File Size (Bytes)"(w328) -> ()
        n109 = local write "Log To File"(w327) -> ()
      }
      frame "Shutdown" {
        n110 = flat-sequence {
          tunnel: w356 -> [w360]
          tunnel: [w360] -> w354
          tunnel: w353 -> [w359]
          tunnel: w352 -> [w358]
          tunnel: [w359] -> w351
          tunnel: [w358] -> w348
          tunnel: [w363] -> w355
          tunnel: w354 -> [w365]
          tunnel: w351 -> [w362]
          tunnel: [w362] -> w350
          tunnel: [w361] -> w349
          tunnel: w348 -> [w361]
          tunnel: w355 -> [_]
          tunnel: [w383] -> w347
          tunnel: w350 -> [w383]
          tunnel: [w382] -> w346
          tunnel: w349 -> [w382]
          frame #0 {
            n111 = call "LJM_Close.vi"("error in"=w358, "Handle"=w359) -> ()  [unwired: 9 in, 1 out]
          }
          frame #1 {
            w364 = u8 0 ("Resolution")
            n112 = local read "# Channels"() -> (w377:i32)
            n113 = local read "Channel Setup"() -> (w380:T1)
            n114 = local read "Data File Prefix"() -> (w374:string)
            n115 = local read "# Scans On Graph"() -> (w376:i32)
            n116 = local read "Disable Scaling*"() -> (w378:bool)
            n117 = local read "Scan Rate (Hz)"() -> (w375:dbl)
            n118 = local read "Max File Size (Bytes)"() -> (w379:i32)
            n119 = local read "Log To File"() -> (w381:bool)
            n120 = global read "LJM logger Globals.vi" "Working Directory"() -> (w372:path)
            n121 = local read "Open Config Name"() -> (w370:string)
            n122 = local read "Open Configs"() -> (w366:T2)
            n123 = Unbundle(w366) -> ("Open Config Device Type"=w369:string, "Open Config Connection Type"=w368:string, "Open Config Identifier"=w367:string)
            n124 = Bundle By Name(cluster=w365, "Data File Prefix"=w374, "Scan Rate (Hz)"=w375, "Graph History"=w376, "# Channels"=w377, "Disable Scaling"=w378, "Max File Size (Bytes)"=w379, "Channel Setup"=w380, "Write To File"=w381) -> (w373:T6)
            n125 = call "LJM logger write open configs.vi"("Working Directory"=w372, "Open Config Filename"=w370, "DeviceType"=w369, "ConnectionType"=w368, "Identifier"=w367) -> ()  [unwired: 10 in, 1 out]
            n126 = local read "Program Config Name"() -> (w371:string)
            n127 = call "LJM logger write program config.vi"("Working Directory"=w372, "filename"=w371, "Program Configs"=w373, "Resolution"=w364, "SettlingFactor"=w364) -> ("error out"=w363:errorcluster)  [unwired: 10 in]
          }
          frame #2 {
            n128 = call "Quit LabVIEW if Executable.vi"() -> ()  [unwired: 1 in]
          }
        }
      }
    }
  }
